vi "VRM_query.vi"() -> ()   [LabVIEW 2016]
uses:
  <instrlib>/Mercury iXX/Public/Libraries/Magnet/Controls/Identifier.ctl
  <instrlib>/Mercury iXX/Public/Controls/Response String.ctl
  <instrlib>/Mercury iXX/Public/Libraries/Magnet/Controls/PSU Actions.ctl
  <instrlib>/Mercury iXX/Public/Controls/Comms Transport Layer.ctl
  <instrlib>/Mercury iXX/Public/Libraries/System/Open/Open System.vi
  <instrlib>/Mercury iXX/Public/Libraries/System/Read/Catalogue (Read).vi
  <instrlib>/Mercury iXX/Public/Libraries/Magnet/Open/Open Magnet Device.vi
  <instrlib>/Mercury iXX/Public/Libraries/Magnet/Signals/Set/Target Field (Set).vi
  <instrlib>/Mercury iXX/Public/Libraries/Magnet/Signals/Set/Target Field Rate (Set).vi
  <instrlib>/Mercury iXX/Public/Libraries/Magnet/Configuration/Set/PSU Action Status (Set).vi
  <instrlib>/Mercury iXX/Public/Libraries/Magnet/Signals/Read/Field (Read).vi
  <instrlib>/Mercury iXX/Public/Libraries/Magnet/Configuration/Read/PSU Action Status (Read).vi
  <instrlib>/Mercury iXX/Mercury iXX.lvlib
  <instrlib>/Mercury iXX/Public/Libraries/Magnet.lvlib
  <instrlib>/Mercury iXX/Public/Libraries/Magnet/Signals/Read/Current (Read).vi
  <instrlib>/Mercury iXX/Public/Libraries/System.lvlib
panel:
  out "PSU Act Stat":T1 caption="PSU Action Status"
  in  "stop":bool
  out "error out":errorcluster
  out "Response 2":T2
  out "Response":T2
  in  "Target Field":dbl format="%#.2f"
  out "Read 1":dbl
  in  "Device ID 3":string(combo)="PSU.M1"
  in  "Device ID 2":string(combo)="GRPY"
  in  "Device ID 1":T3="GRPZ"
  out "Read 2":dbl format="%_15p"
  out "Read 3":dbl format="%_10p"
  out "Devices":string[](array[string])
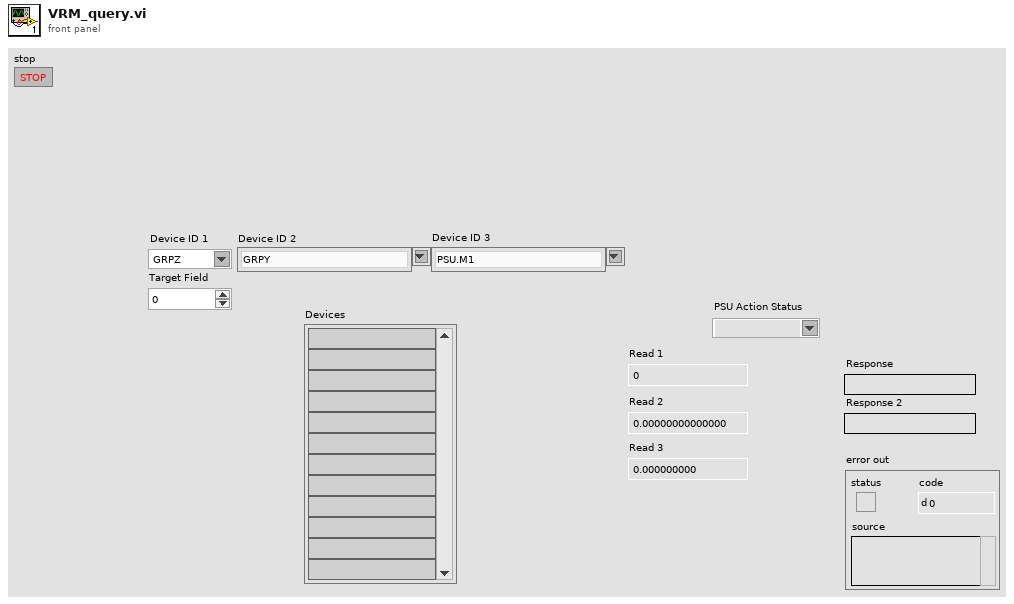
[diagram p1: front panel]
types:
  T1 = typedef "Mercury iXX.lvlib/Magnet.lvlib/PSU Actions.ctl" = string
  T2 = typedef "Mercury iXX.lvlib/Response String.ctl" = string
  T3 = typedef "Mercury iXX.lvlib/Magnet.lvlib/Identifier.ctl" = string
  T4 = typedef "Mercury iXX.lvlib/Comms Transport Layer.ctl" = enum16{"Ethernet TCP/IP", "USB", "ISOBus - RS-232", "GPIB"}
  T5 = typedef "Mercury iXX.lvlib/Mercury Reference.ctl" = cluster{"Comms":refnum<visa-resource-name>, "Device ID":string[], "Comms Layer":T4, "Command":string, "Query reference":T6}
  T6 = typedef "Mercury iXX.lvlib/Query Dynamic Reference.ctl" = refnum<vi>
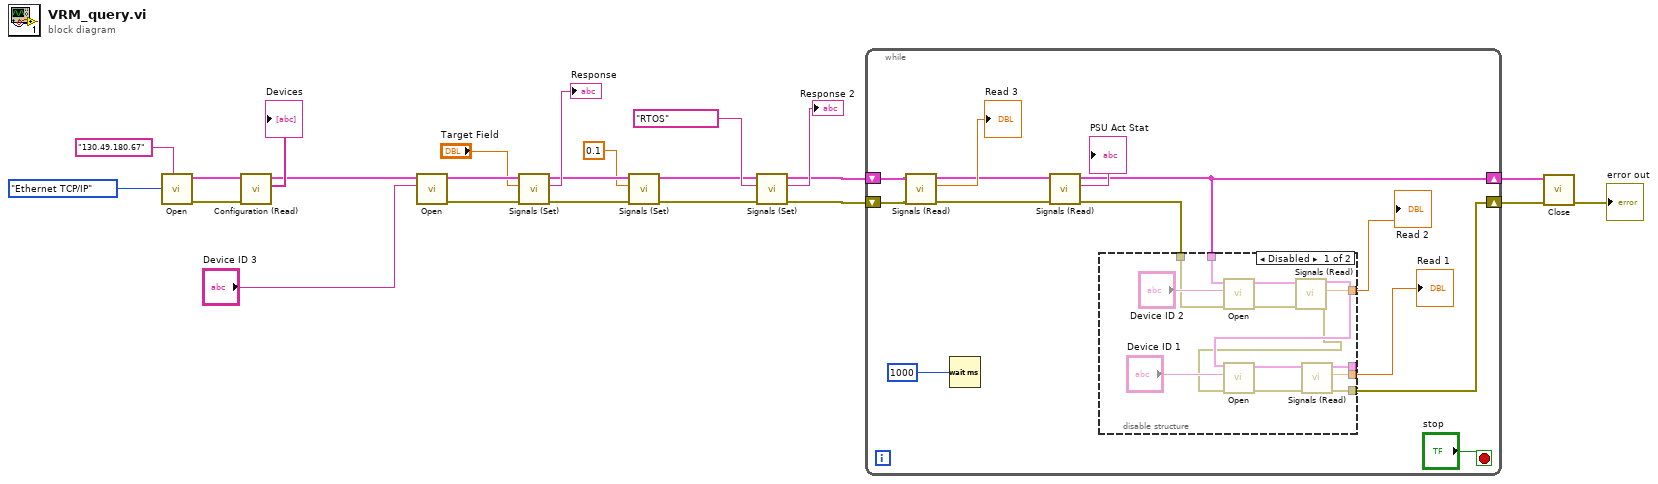
[diagram p0: block diagram]
diagram:
  n1 = call-poly <instrlib>:"Open.vi"("IP Address"="130.49.180.67", "Comms Layer"=Comms_Transport_Layer."Ethernet TCP/IP") -> ("error out"=w20:errorcluster, "Mercury Reference Out"=w21:T5)  [unwired: 5 in, 3 out]
  n2 = call-poly <instrlib>:"Configuration (Read).vi"("error in"=w20, "Mercury Reference In"=w21) -> ("Devices"=→"Devices":string[], "Mercury Reference Out"=w17:T5)  [unwired: 6 in, 2 out]
  n3 = call-poly <instrlib>:"Open.vi"("Device Identifier"="Device ID 3", "Mercury Reference In"=w17) -> ("error out"=w14:errorcluster, "Mercury Reference Out"=w16:T5)  [unwired: 8 in]
  n4 = call-poly <instrlib>:"Signals (Set).vi"("error in"=w14, "Target Field"="Target Field", "Mercury Reference In"=w16) -> ("error out"=w3:errorcluster, "Response"=→"Response":T2, "Mercury Reference Out"=w7:T5)  [unwired: 5 in, 1 out]
  n5 = call-poly <instrlib>:"Signals (Set).vi"("error in"=w3, "Target Field Rate"=0.1 ("Target Field"), "Mercury Reference In"=w7) -> ("error out"=w4:errorcluster, "Mercury Reference Out"=w5:T5)  [unwired: 5 in, 2 out]
  n6 = call-poly <instrlib>:"Signals (Set).vi"("error in"=w4, "PSU Act Stat"=T1 "RTOS", "Mercury Reference In"=w5) -> ("error out"=w8:errorcluster, "Response"=→"Response 2":T2, "Mercury Reference Out"=w11:T5)  [unwired: 5 in, 1 out]
  n7 = while {
    shift-right: [w24] -> w2
    shift-left: w11 -> [w33]
    shift-right: [w28] -> w1
    shift-left: w8 -> [w32]
    stop <- "stop" stop-if-true
    n8 = call-poly "Signals (Read).vi"("error in"=w32, "Mercury Reference In"=w33) -> ("error out"=w30:errorcluster, "Field"=→"Read 3":dbl, "Mercury Reference Out"=w29:T5)  [unwired: 5 in, 2 out]
    n9 = Wait (ms)(milliseconds to wait=u32 1000) -> ()  [unwired: 1 out]
    n10 = call-poly "Signals (Read).vi"("error in"=w30, "Mercury Reference In"=w29) -> ("error out"=w27:errorcluster, "PSU Act Stat"=→"PSU Act Stat":T1, "Mercury Reference Out"=w24:T5)  [unwired: 6 in, 1 out]
    n11 = disable-structure shown="Disabled" {
      disable-tunnel: [w48 _] -> w36
      disable-tunnel: [w44 _] -> w34
      disable-tunnel: w24 -> [w42 _]
      disable-tunnel: [w40 _] -> _
      disable-tunnel: [w39 _] -> w28
      disable-tunnel: w27 -> [w37 _]
      frame Disabled {
        n12 = call-poly <instrlib>:"Open.vi"("error in (no error)"=w37, "Device Identifier"="Device ID 2", "Mercury Reference In"=w42) -> ("error out"=w49:errorcluster, "Mercury Reference Out"=w50:T5)  [unwired: 7 in]
        n13 = call-poly "Signals (Read).vi"("error in"=w49, "Mercury Reference In"=w50) -> ("error out"=w38:errorcluster, "Current"=w48:dbl, "Mercury Reference Out"=w41:T5)  [unwired: 5 in, 2 out]
        n14 = call-poly <instrlib>:"Open.vi"("error in (no error)"=w38, "Device Identifier"="Device ID 1", "Mercury Reference In"=w41) -> ("error out"=w43:errorcluster, "Mercury Reference Out"=w45:T5)  [unwired: 7 in]
        n15 = call-poly "Signals (Read).vi"("error in"=w43, "Mercury Reference In"=w45) -> ("error out"=w39:errorcluster, "Current"=w44:dbl, "Mercury Reference Out"=w40:T5)  [unwired: 5 in, 2 out]
      }
      frame Enabled {
      }
    }
    "Read 2" <- w36
    "Read 1" <- w34
  }
  n16 = call <instrlib>:"Close.vi"("error in (no error)"=w1, "Mercury Reference"=w2) -> ("error out"=→"error out":errorcluster)  [unwired: 9 in]
